vi "p1.vi"() -> ()   [LabVIEW 2025, in "d8.lvlib"]
uses:
  d8.lvlib
  1b063c04-a246-46ef-9c2d-d8fe64587413.vi
  lv2025-aoc/AOC/AOC.lvlib
panel:
  in  "Example":string="RL\n\nAAA = (BBB, CCC)\nBBB = (DDD, EEE)\nCCC = (ZZZ, GGG)\nDDD = (DDD, DDD)\nEEE = (EEE, EEE)\nGGG = (GGG, GGG)\nZZZ = (ZZZ, ZZZ)"
  in  "Example":bool
  out "Answer":i32=12169
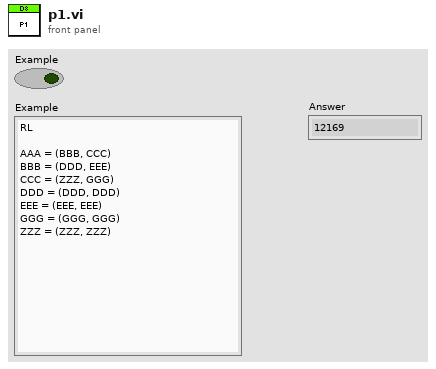
[diagram p1: front panel]
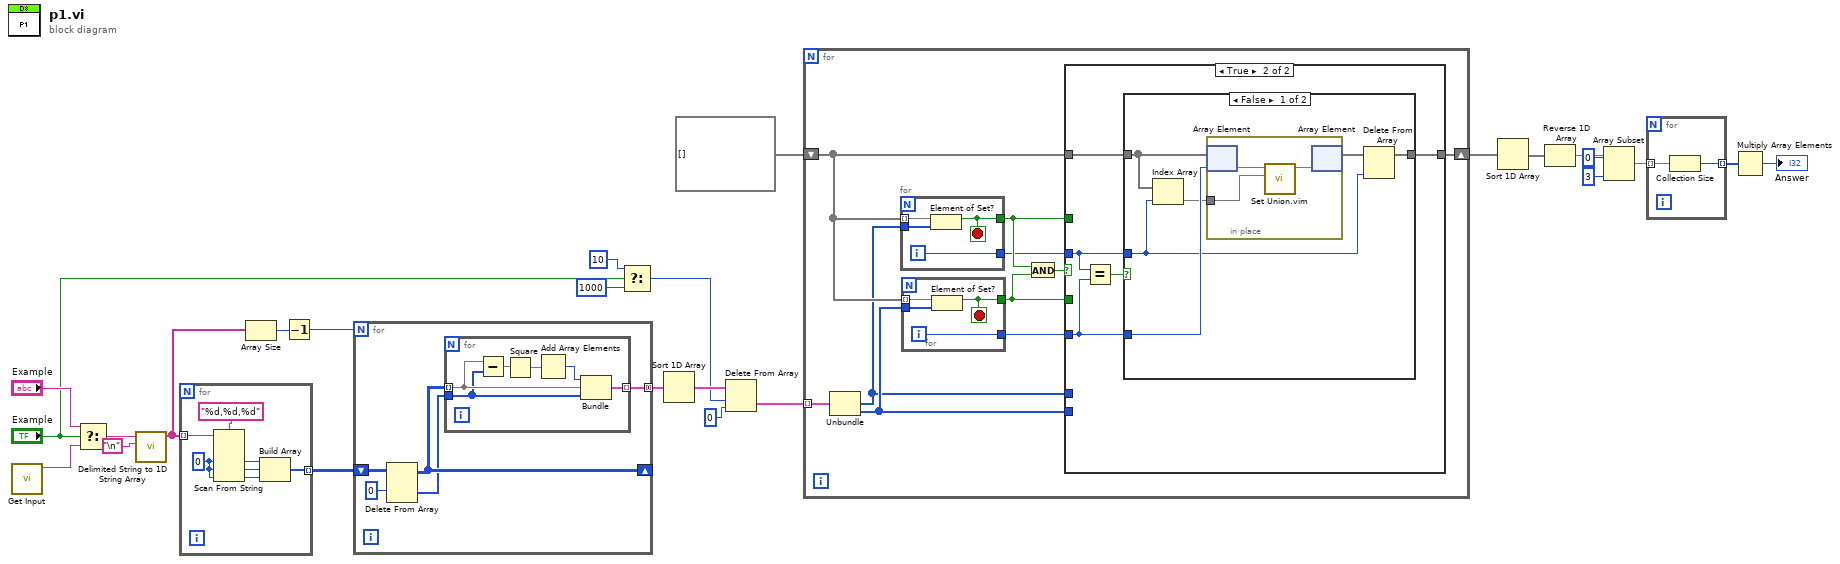
[diagram p0: block diagram]
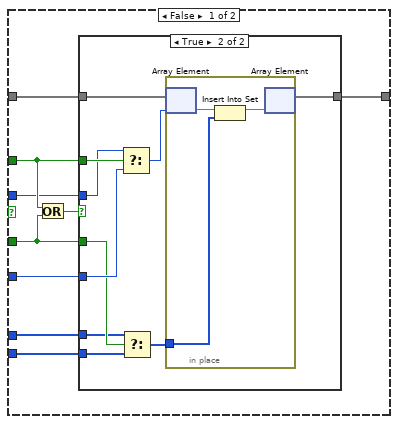
[diagram p2: hidden frame]
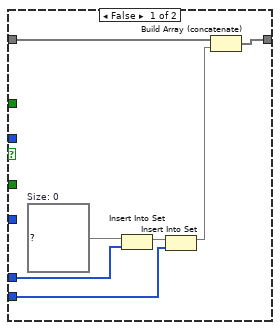
[diagram p3: hidden frame]
diagram:
  n1 = call "Get Input.vi"() -> ("Input"=w25:string)  [unwired: 11 in]
  n2 = Select(t="Example", s="Example", f=w25) -> (s? t:f=w24:string)
  n3 = call <vilib>:"Delimited String to 1D String Array.vi"("delimiter"="\n", "delimited string"=w24) -> ("string array"=w21:string[])  [unwired: 9 in]
  n4 = for {
    tunnel: w21 -> [w32] mode=indexing
    tunnel: [w27] -> w20 mode=indexing
    w26 = i64 0 ("default value 14")
    n5 = Scan From String(format string="%d,%d,%d", input string=w32, default 1=w26, default 2=w26, default 3=w26) -> (output 1=w30:i64, output 2=w29:i64, output 3=w28:i64)  [unwired: 2 in, 3 out]
    n6 = Build Array(w30, w29, w28) -> (w27:i64[])
  }
  n7 = Array Size(array=w21) -> (size(s)=w19:i32)
  n8 = Decrement(x=w19) -> (x-1=w6:i32)
  n9 = for {
    N: w6 -> [_]
    shift-right: [w35] -> _
    shift-left: w20 -> [w37]
    tunnel: [w33] -> w18 mode=concatenating
    n10 = Delete From Array(array=w37, index (row)=0) -> (deleted portion=w34:i64[], array with subset deleted=w35:i64[][])  [unwired: 2 in]
    n11 = for {
      tunnel: w35 -> [w43] mode=indexing
      tunnel: w34 -> [w42]
      tunnel: [w38] -> w33 mode=indexing
      n12 = Subtract(x=w43, y=w42) -> (x-y=w41:i64[])
      n13 = Square(x=w41) -> (x^2=w40:i64[])
      n14 = Add Array Elements(numeric array=w40) -> (sum=w39:i64)
      n15 = Bundle("default value 14"=w39, w43, w42) -> (w38:cluster{"default value 14":i64, i64[], i64[]})  [unwired: 1 in]
    }
  }
  n16 = Select(t=10 ("length"), s="Example", f=1000) -> (s? t:f=w4:i32)
  n17 = Sort 1D Array(array=w18) -> (sorted array=w17:cluster{"default value 14":i64, i64[], i64[]}[])
  n18 = Delete From Array(array=w17, length=w4, index=0) -> (deleted portion=w14:cluster{"default value 14":i64, i64[], i64[]}[])  [unwired: 1 out]
  n19 = for {
    shift-right: [w46] -> w13
    shift-left: set{i64[]}[] [] -> [w47]
    tunnel: w14 -> [w53] mode=indexing
    n20 = Unbundle(w53) -> (w44:i64[], w45:i64[])  [unwired: 1 out]
    n21 = for {
      tunnel: w44 -> [w104]
      tunnel: w47 -> [w105] mode=indexing
      tunnel: [w103] -> w51
      tunnel: [w102] -> w49
      i -> [w102]
      stop <- w103 stop-if-true
      n22 = Element of Set?(10:w104, 11:w105) -> (3:w103:bool)
    }
    n23 = for {
      tunnel: w45 -> [w100]
      tunnel: w47 -> [w101] mode=indexing
      tunnel: [w99] -> w50
      tunnel: [w98] -> w48
      i -> [w98]
      stop <- w99 stop-if-true
      n24 = Element of Set?(10:w100, 11:w101) -> (3:w99:bool)
    }
    n25 = And(x=w51, y=w50) -> (x .and. y?=w52:bool)
    n26 = case shown="True" w52 {
      tunnel: w51 -> [w61 _]
      tunnel: w50 -> [w57 _]
      tunnel: w49 -> [w59 w86]
      tunnel: w48 -> [w60 w85]
      tunnel: w47 -> [w58 w84]
      tunnel: [w54 w83] -> w46
      tunnel: w45 -> [w55 _]
      tunnel: w44 -> [w56 _]
      frame False {
        n27 = Or(x=w61, y=w57) -> (x .or. y?=w62:bool)
        n28 = case shown="True" w62 {
          tunnel: w61 -> [_ w79]
          tunnel: w60 -> [_ w78]
          tunnel: w59 -> [_ w77]
          tunnel: w58 -> [w69 w76]
          tunnel: w57 -> [_ w74]
          tunnel: w56 -> [w64 w73]
          tunnel: w55 -> [w63 w72]
          tunnel: [w68 w70] -> w54
          frame False {
            w65 = set{i64[]} {}  # Size: 0
            n29 = Insert Into Set(10:w64, 11:w65) -> (3:w66:set{i64[]})  [unwired: 1 out]
            n30 = Insert Into Set(10:w63, 11:w66) -> (3:w67:set{i64[]})  [unwired: 1 out]
            n31 = Build Array (concatenate)(w69, w67) -> (w68:set{i64[]}[])
          }
          frame True {
            n32 = Select(t=w77, s=w79, f=w78) -> (s? t:f=w75:i32)
            n33 = Select(t=w73, s=w74, f=w72) -> (s? t:f=w71:i64[])
            n34 = in-place {
              in-place-border: w71 -> [w80]
              n35 = in-place-array #1(w76, w75) -> (w82:set{i64[]})
              n36 = Insert Into Set(10:w80, 11:w82) -> (3:w81:set{i64[]})  [unwired: 1 out]
              n37 = in-place-array #1(w81) -> (w70:set{i64[]}[])  [unwired: 1 out]
            }
          }
        }
      }
      frame True {
        n38 = Equal?(x=w86, y=w85) -> (x = y?=w87:bool)
        n39 = case shown="False" w87 {
          tunnel: w86 -> [w88 _]
          tunnel: w85 -> [w93 _]
          tunnel: w84 -> [w91 w97]
          tunnel: [w89 w97] -> w83
          frame False {
            n40 = Index Array(array=w91, index=w88) -> (element=w90:set{i64[]})
            n41 = in-place {
              in-place-border: w90 -> [w95]
              n42 = in-place-array #2(w91, w93) -> (w96:set{i64[]})
              n43 = call "Set Union.vim"("set 2"=w95, "set 1"=w96) -> ("union"=w94:set{i64[]})  [unwired: 9 in]
              n44 = in-place-array #2(w94) -> (w92:set{i64[]}[])  [unwired: 1 out]
            }
            n45 = Delete From Array(array=w92, index=w88) -> (array with subset deleted=w89:set{i64[]}[])  [unwired: 1 in, 1 out]
          }
          frame True {
          }
        }
      }
    }
  }
  n46 = Sort 1D Array(array=w13) -> (sorted array=w12:set{i64[]}[])
  n47 = Reverse 1D Array(array=w12) -> (reversed array=w11:set{i64[]}[])
  n48 = Array Subset(array=w11, index=0, length=3) -> (w9:set{i64[]}[])
  n49 = for {
    tunnel: w9 -> [w107] mode=indexing
    tunnel: [w106] -> w8 mode=indexing
    n50 = Collection Size(1:w107) -> (0:w106:i32)
  }
  n51 = Multiply Array Elements(1:w8) -> (0:→"Answer":i32)
